vi "Process.vi"(8 "error in":errorcluster, 11 "Qbus in":refnum<class "Qbus.lvclass">) -> (0 "error out":errorcluster)   [LabVIEW 2021, in "AnalogGenerationProcess.lvlib"]
uses:
  AnalogGenerationProcess.lvlib
  <vilib>/addons/Qbus/Qbus.lvclass
  controls/state.ctl
  <vilib>/addons/_NISVFA/_Generation/Signal Generation/SV Signal/SV Signal.lvclass
  controls/generation status.ctl
  <vilib>/addons/_NISVFA/_Generation/Signal Generation/SV Signal/sv_System Timing Model.ctl
  controls/analog generation settings.ctl
  controls/analog output settings.ctl
  controls/terminal configuration.ctl
  controls/signal settings.ctl
  controls/signal type.ctl
  controls/sine wave properties.ctl
  <vilib>/DAQmx/write.llb/DAQmx Write (Analog Wfm 1Chan NSamp).vi
  <vilib>/addons/_NISVFA/_Generation/Signal Generation/SV Sinusoid/SV Sinusoid.lvclass
  C:/Program Files/National Instruments/LabVIEW 2021/vi.lib/addons/_NISVFA/_Generation/Signal Generation/SV Signal/SV Signal.lvclass
  <vilib>/addons/_NISVFA/_Generation/Signal Generation/SV Sinusoid/Configure Sine.vi
  <vilib>/addons/_NISVFA/_Generation/Signal Generation/SV Signal/Write Sample Rate.vi
  <vilib>/addons/_NISVFA/_Generation/Signal Generation/SV Signal/Write System Timing Model.vi
  <vilib>/addons/_NISVFA/_Generation/Signal Generation/SV Signal/Write Ramp Parameters.vi
  <vilib>/DAQmx/miscellaneous.llb/DAQmx Fill In Error Info.vi
  subVIs/utility/AudioGenUtility.lvlib
  shared/logger process/EventLoggerProcess.lvlib
  controls/AudioGenTypeDefs.lvlib
  C:/Program Files/National Instruments/LabVIEW 2021/vi.lib/addons/_NISVFA/_Generation/Signal Generation/SV Function/SV Function.lvclass
  C:/Program Files/National Instruments/LabVIEW 2021/vi.lib/addons/_NISVFA/_Generation/Signal Generation/SV Sinusoid/SV Sinusoid.lvclass
  controls/update signal settings.ctl
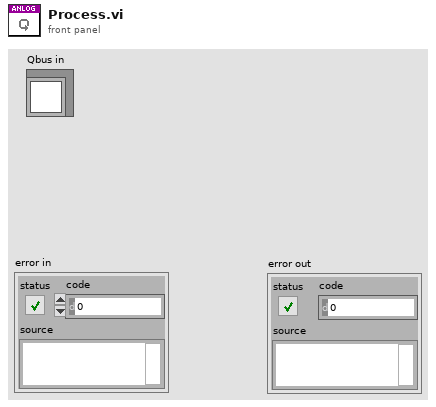
[diagram p1: front panel]
types:
  T1 = typedef "AnalogGenerationProcess.lvlib/state.ctl" = cluster{"DAQmx task":refnum<k21>, "signal configuration":refnum<class "SV Signal.lvclass">, "status":T2}
  T2 = typedef "AudioGenTypeDefs.lvlib/generation status.ctl" = enum16{"Idle", "Committed", "Active"}
  T3 = typedef "AudioGenTypeDefs.lvlib/analog generation settings.ctl" = cluster{"channel list":string, "output settings":T4, "signal settings":T6}
  T4 = typedef "AudioGenTypeDefs.lvlib/analog output settings.ctl" = cluster{"output rate":dbl, "range":dbl, "terminal configuration":T5, "output impedance":dbl, "common mode offset":dbl, "pure tone mode":bool}
  T5 = typedef "AudioGenTypeDefs.lvlib/terminal configuration.ctl" = enum32{"Default", "RSE", "Differential", "Pseudodifferential"}
  T6 = typedef "AudioGenTypeDefs.lvlib/signal settings.ctl" = cluster{"signal type":T7, "properties":string}
  T7 = typedef "AudioGenTypeDefs.lvlib/signal type.ctl" = enum16{"Sine", "Square", "Triangle", "White Noise", "Pink Noise", "Periodic Random Noise"}
  T8 = cluster{"profile":enum16{"Linear", "Half cosine"}, "durations [s]":cluster{"ramp-up":dbl, "transition":dbl, "ramp-down":dbl}}
  T9 = typedef "AudioGenTypeDefs.lvlib/sine wave properties.ctl" = cluster{"frequency":dbl, "amplitude":dbl, "phase":dbl}
  T10 = typedef "AudioGenTypeDefs.lvlib/update signal settings.ctl" = cluster{"frequency":dbl, "gain":dbl}
  T11 = typedef "SV Signal.lvclass/sv_System Timing Model.ctl" = i64
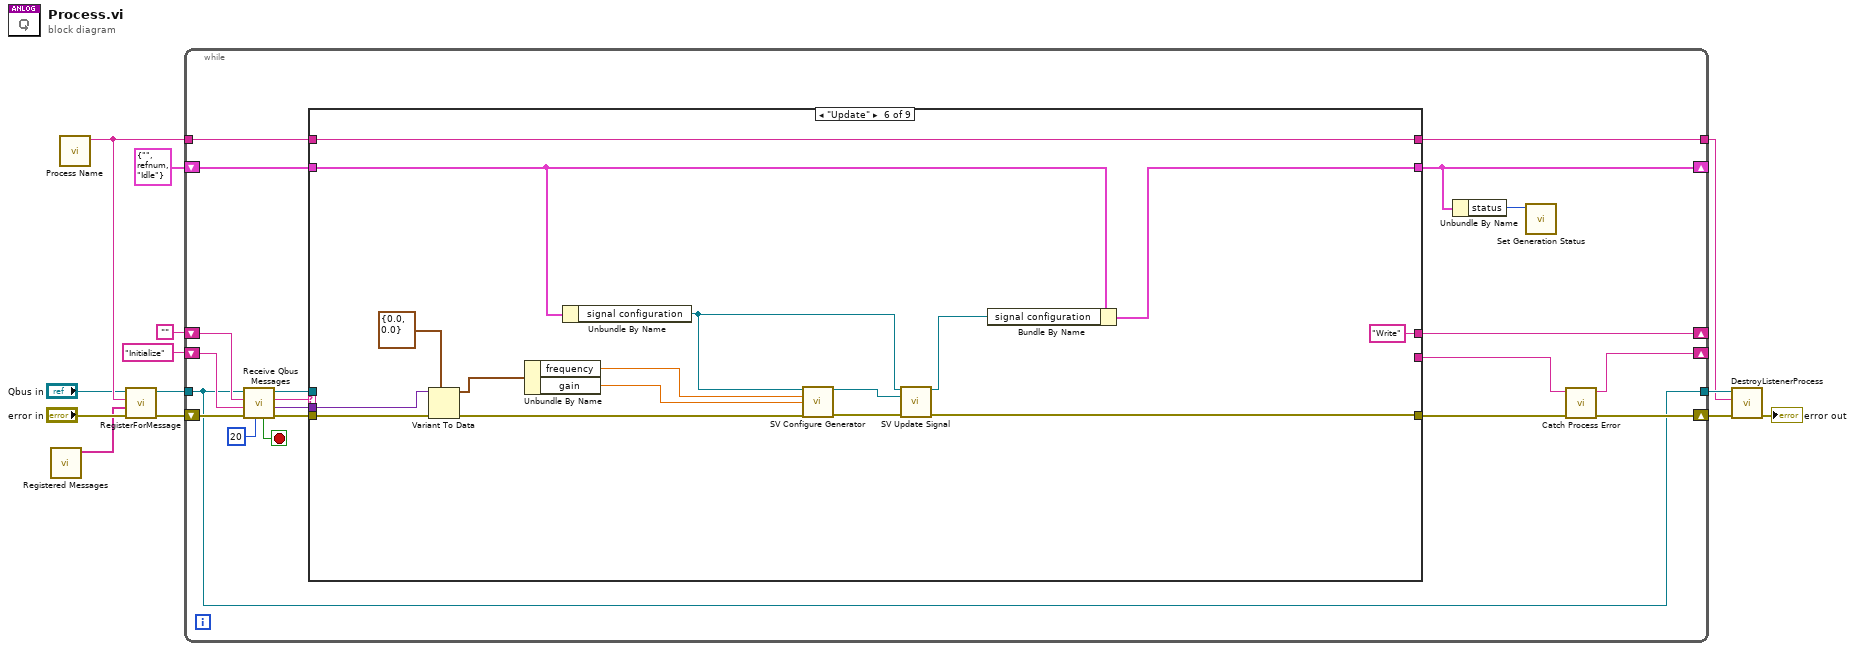
[diagram p0: block diagram]
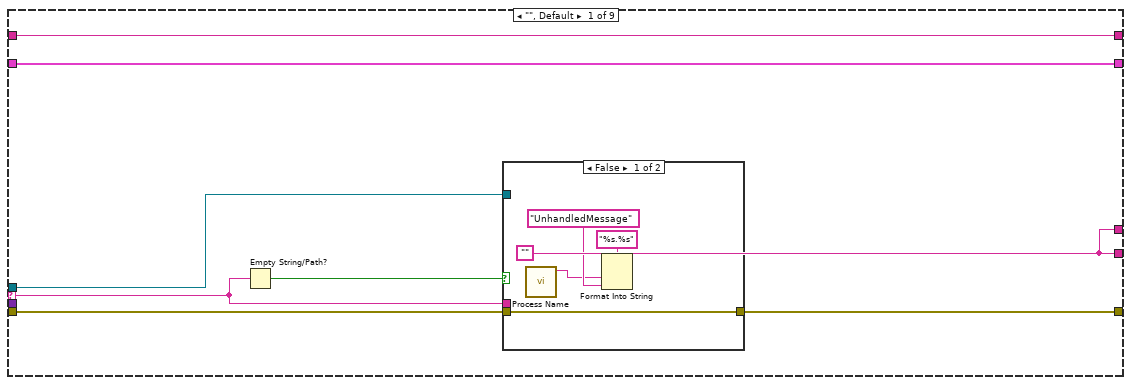
[diagram p2: hidden frame]
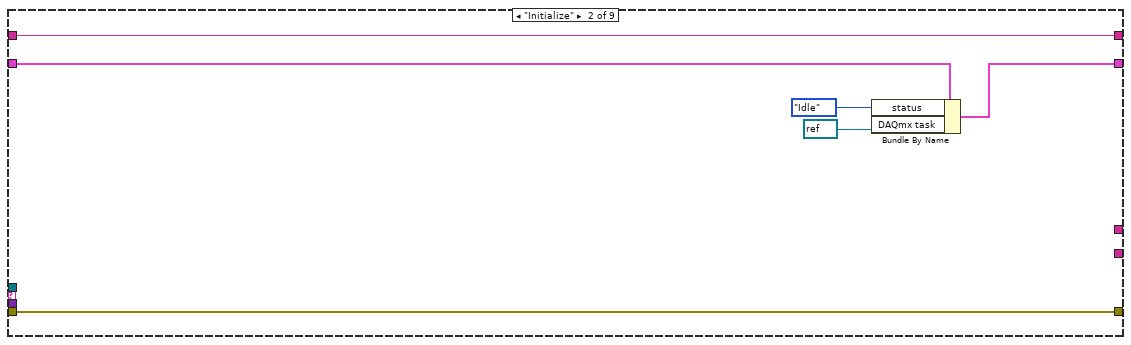
[diagram p4: hidden frame]
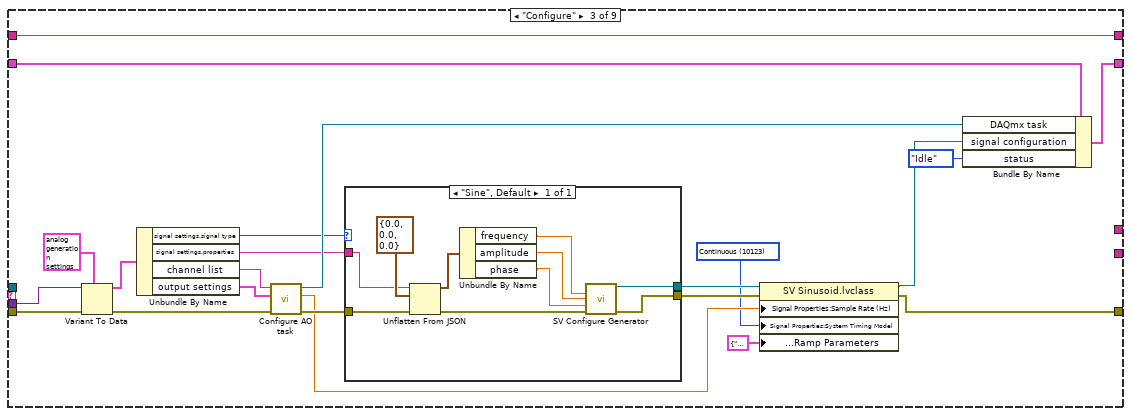
[diagram p5: hidden frame]
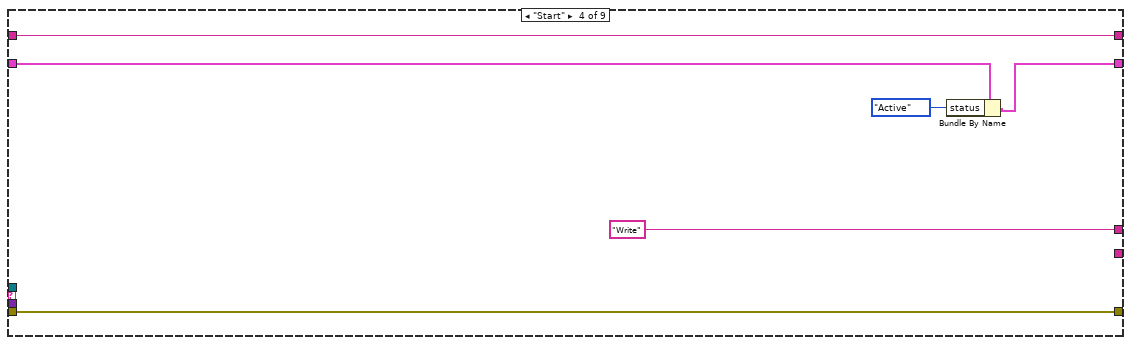
[diagram p6: hidden frame]
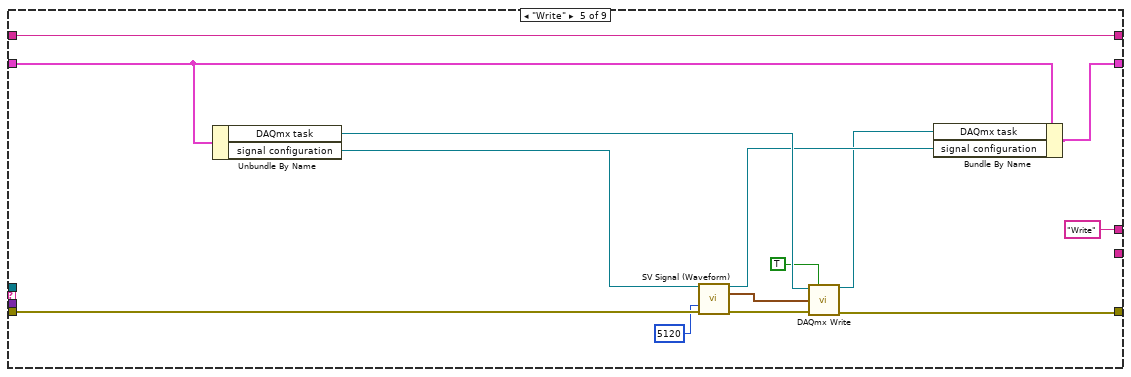
[diagram p7: hidden frame]
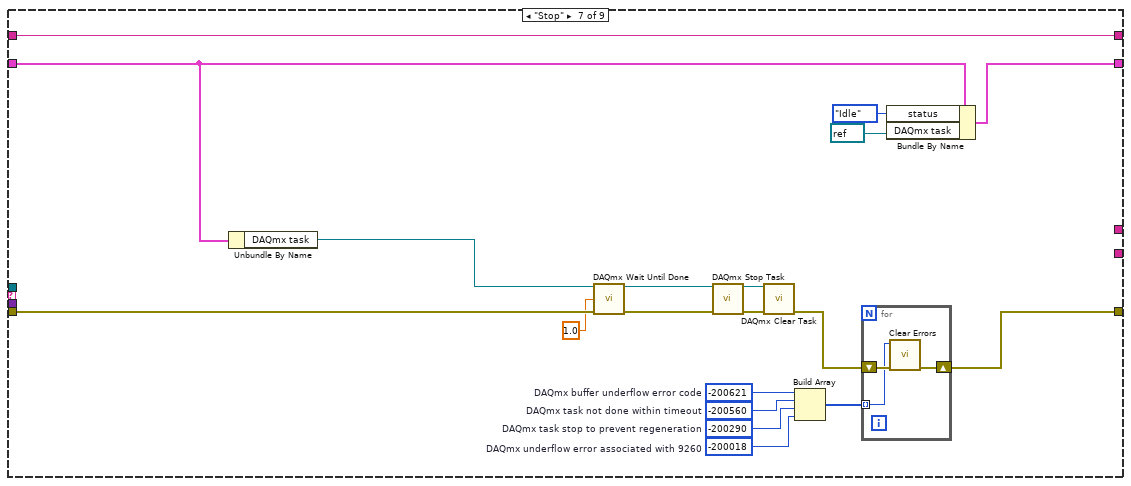
[diagram p8: hidden frame]
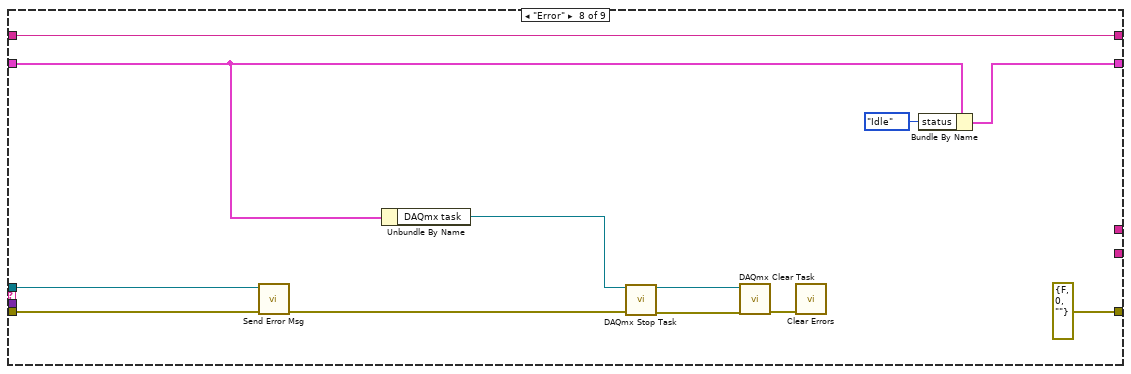
[diagram p9: hidden frame]
diagram:
  n1 = call "Registered Messages.vi"() -> ("registered messages"=w6:string[])  [unwired: 11 in]
  n2 = call "Process Name.vi"() -> ("process name"=w9:string)  [unwired: 11 in]
  n3 = call <vilib>:"RegisterForMessage.vi"("error in (no error)"="error in", "message names"=w6, "process name"=w9, "Qbus in"="Qbus in") -> ("error in (no error)"=w12:errorcluster, "Qbus out"=w13:refnum<class "Qbus.lvclass">)  [unwired: 6 in]
  n4 = while {
    shift-right: [w20] -> _
    shift-left: "" -> [w32]
    tunnel: w13 -> [w16]
    tunnel: w9 -> [w18]
    tunnel: [w16] -> w4
    tunnel: [w22] -> w2
    shift-right: [w26] -> _
    shift-left: "Initialize" -> [w28]
    shift-right: [w27] -> w5
    shift-left: w12 -> [w25]
    shift-right: [w15] -> _
    shift-left: T1 {"DAQmx task"="", "signal configuration"=refnum, "status"=enum."Idle"} ("state") -> [w17]
    stop <- w33 stop-if-true
    n5 = call "Receive Qbus Messages.vi"("timeout(ms)"=20 ("milliseconds to wait"), "error in (no error)"=w25, "priority action"=w28, "default action"=w32, "Qbus in"=w16) -> ("error out"=w31:errorcluster, "message value"=w29:variant, "action"=w24:string, "Qbus out"=w30:refnum<class "Qbus.lvclass">, "exit"=w33:bool)  [unwired: 2 in]
    n6 = case shown="\"Update\"" w24 {
      selector: w24 -> [w38 _ _ _ _ _ _ _ _]
      tunnel: w31 -> [w40 w52 w61 w90 w103 w110 w138 w153 w157]
      tunnel: w30 -> [w36 _ _ _ _ _ _ w152 _]
      tunnel: [w39 w52 w67 w90 w98 w116 w126 errorcluster {"status"=FALSE, "code"=0, "source"=""} ("error out") w157] -> w19
      tunnel: w29 -> [_ _ w62 _ _ w108 _ _ _]
      tunnel: [w41 w51 w74 w89 w104 w120 w139 w154 w156] -> w22
      tunnel: w18 -> [w41 w51 w74 w89 w104 w120 w139 w154 w156]
      tunnel: [w35 _ _ _ _ _ _ _ _] -> w21
      tunnel: [w35 _ _ "Write" "Write" "Write" _ _ _] -> w20
      tunnel: w17 -> [w34 w50 w73 w88 w93 w114 w134 w145 w155]
      tunnel: [w34 w49 w72 w86 w92 w113 w133 w144 w155] -> w15
      frame "", Default {
        w35 = ""
        n7 = Empty String/Path?(string/path=w38) -> (empty?=w37:bool)
        n8 = case shown="False" w37 {
          tunnel: [w42 w46] -> w39
          tunnel: w40 -> [w42 w46]
          tunnel: w38 -> [_ _]
          tunnel: w36 -> [_ _]
          frame False {
            n9 = call "Process Name.vi"() -> ("process name"=w43:string)  [unwired: 11 in]
            n10 = Format Into String(format string="%s.%s", w43, "UnhandledMessage" ("ProcessName")) -> ()  [unwired: 2 in, 2 out]
          }
          frame True {
          }
        }
      }
      frame "Initialize" {
        n11 = Bundle By Name(cluster=w50, "status"=enum16{"Idle", "Committed", "Active"}."Idle", "DAQmx task"=refnum<k21> refnum) -> (w49:T1)
      }
      frame "Configure" {
        w65 = T11 10123 items=["Finite"=10178, "-"=-1, "Continuous"=10123, "-"=-2, "Settled"=110123, "Averaged"=210123, "Discrete Sweep"=310123, "Continuous Sweep"=410123] ("System Timing Model")
        n12 = Variant To Data(error in=w61, type=T3 {"channel list"="", "output settings"={"output rate"=0.0, "range"=0.0, "terminal configuration"=enum."Pseudodifferential", "output impedance"=0.0, "common mode offset"=0.0, "pure tone mode"=FALSE}, "signal settings"={"signal type"=enum."Sine", "properties"=""}} ("analog generation"), Variant=w62) -> (data=w59:T3, error out=w58:errorcluster)
        n13 = Unbundle By Name(w59) -> ("signal settings.signal type"=w57:T7, "signal settings.properties"=w56:string, "channel list"=w55:string, "output settings"=w54:T4)
        n14 = call "Configure AO task.vi"("error in (no error)"=w58, "analog generation"=w54, "physical channels"=w55) -> ("error out"=w71:errorcluster, "actual sample rate"=w66:dbl, "task out"=w63:refnum<k21>)  [unwired: 6 in]
        n15 = case shown="\"Sine\", Default" w57 {
          tunnel: w71 -> [w82]
          tunnel: [w84] -> w70
          tunnel: [w83] -> w69
          tunnel: w56 -> [w79]
          frame "Sine", Default {
            n16 = Unflatten From JSON(JSON string=w79, type and defaults=T9 {"frequency"=0.0, "amplitude"=0.0, "phase"=0.0} ("sine wave properties"), error in (no error)=w82) -> (value=w78:T9, error out=w81:errorcluster)  [unwired: 4 in]
            n17 = Unbundle By Name(w78) -> ("frequency"=w77:dbl, "amplitude"=w76:dbl, "phase"=w75:dbl)
            n18 = call-poly <vilib>:"SV Configure Generator.vi"("frequency (Hz)"=w77, "amplitude"=w76, "phase (deg)"=w75, "error in (no error)"=w81) -> ("signal configuration"=w84:refnum<class "SV Sinusoid.lvclass">, "error out"=w83:errorcluster)  [unwired: 10 in]
          }
        }
        n19 = property class="SV Sinusoid.lvclass"(reference=w70, error in=w69, "Signal Properties:Sample Rate (Hz)"=w66, "Signal Properties:System Timing Model"=w65, "Signal Properties:Ramps:Ramp Parameters"=T8 {"profile"=enum."Half cosine", "durations [s]"={"ramp-up"=0.01, "transition"=0.01, "ramp-down"=0.01}} ("Ramp Parameters:All Elements")) -> (reference out=w68:refnum<class "SV Sinusoid.lvclass">, error out=w67:errorcluster)
        n20 = Bundle By Name(cluster=w73, "DAQmx task"=w63, "signal configuration"=w68, "status"=generation_status."Idle") -> (w72:T1)
      }
      frame "Start" {
        n21 = Bundle By Name(cluster=w88, "status"=enum16{"Idle", "Committed", "Active"}."Active") -> (w86:T1)
      }
      frame "Write" {
        n22 = Unbundle By Name(w93) -> ("DAQmx task"=w100:refnum<k21>, "signal configuration"=w102:refnum<class "SV Signal.lvclass">)
        n23 = call-dynamic "SV Signal (Waveform).vi"("signal configuration"=w102, "samples"=5120, "error in (no error)"=w103) -> ("signal configuration"=w95:refnum<class "SV Signal.lvclass">, "output waveform"=w99:waveform(dbl), "error out"=w101:errorcluster)  [unwired: 7 in, 3 out]
        n24 = call-poly <vilib>:"DAQmx Write.vi"("task/channels in"=w100, "auto start"=TRUE, "data"=w99, "error in"=w101) -> ("task out"=w94:refnum<k21>, "error out"=w98:errorcluster)  [unwired: 9 in, 1 out]
        n25 = Bundle By Name(cluster=w93, "DAQmx task"=w94, "signal configuration"=w95) -> (w92:T1)
      }
      frame "Update" {
        n26 = Variant To Data(error in=w110, type=T10 {"frequency"=0.0, "gain"=0.0} ("signal update setting"), Variant=w108) -> (data=w107:T10, error out=w109:errorcluster)
        n27 = Unbundle By Name(w107) -> ("frequency"=w106:dbl, "gain"=w105:dbl)
        n28 = Unbundle By Name(w114) -> ("signal configuration"=w119:refnum<class "SV Signal.lvclass">)
        n29 = call-poly <vilib>:"SV Configure Generator.vi"("template configuration"=w119, "frequency (Hz)"=w106, "amplitude"=w105, "error in (no error)"=w109) -> ("signal configuration"=w118:refnum<class "SV Sinusoid.lvclass">, "error out"=w117:errorcluster)  [unwired: 10 in]
        n30 = call-dynamic "SV Update Signal.vi"("current configuration"=w119, "new configuration"=w118, "error in"=w117) -> ("updated configuration"=w115:refnum<class "SV Sinusoid.lvclass">, "error out"=w116:errorcluster)  [unwired: 11 in]
        n31 = Bundle By Name(cluster=w114, "signal configuration"=w115) -> (w113:T1)
      }
      frame "Stop" {
        w129 = -200018  # DAQmx underflow error associated with 9260
        w130 = -200290  # DAQmx task stop to prevent regeneration
        w131 = -200560  # DAQmx task not done within timeout
        w132 = -200621  # DAQmx buffer underflow error code
        n32 = Unbundle By Name(w134) -> ("DAQmx task"=w137:refnum<k21>)
        n33 = call <vilib>:"DAQmx Wait Until Done.vi"("task/channels in"=w137, "timeout (sec)"=1.0, "error in"=w138) -> ("task out"=w136:refnum<k21>, "error out"=w127:errorcluster)  [unwired: 11 in]
        n34 = call <vilib>:"DAQmx Stop Task.vi"("task/channels in"=w136, "error in"=w127) -> ("task out"=w124:refnum<k21>, "error out"=w123:errorcluster)  [unwired: 12 in]
        n35 = call <vilib>:"DAQmx Clear Task.vi"("task in"=w124, "error in"=w123) -> ("error out"=w122:errorcluster)  [unwired: 13 in]
        n36 = Build Array(w132, w131, w130, w129) -> (w128:i32[])
        n37 = for {
          shift-right: [w141] -> w126
          shift-left: w122 -> [w142]
          tunnel: w128 -> [w140] mode=indexing
          n38 = call <vilib>:"Clear Errors.vi"("error in (no error)"=w142, "specific error code to clear (0: all)"=w140) -> ("error out"=w141:errorcluster)  [unwired: 4 in, 1 out]
        }
        n39 = Bundle By Name(cluster=w134, "status"=generation_status."Idle", "DAQmx task"=refnum<k21> refnum) -> (w133:T1)
      }
      frame "Error" {
        n40 = call "Send Error Msg.vi"("error in"=w153, "Qbus in"=w152) -> ("error out"=w150:errorcluster)  [unwired: 8 in, 1 out]
        n41 = Unbundle By Name(w145) -> ("DAQmx task"=w149:refnum<k21>)
        n42 = call <vilib>:"DAQmx Stop Task.vi"("task/channels in"=w149, "error in"=w150) -> ("task out"=w148:refnum<k21>, "error out"=w147:errorcluster)  [unwired: 12 in]
        n43 = call <vilib>:"DAQmx Clear Task.vi"("task in"=w148, "error in"=w147) -> ("error out"=w146:errorcluster)  [unwired: 13 in]
        n44 = call <vilib>:"Clear Errors.vi"("error in (no error)"=w146) -> ()  [unwired: 5 in, 2 out]
        n45 = Bundle By Name(cluster=w145, "status"=generation_status."Idle") -> (w144:T1)
      }
      frame "Exit" {
      }
    }
    n46 = Unbundle By Name(w15) -> ("status"=w14:T2)
    n47 = call "Set Generation Status.vi"("status"=w14) -> ()  [unwired: 10 in, 1 out]
    n48 = call "Catch Process Error.vi"("error in (no error)"=w19, "priority action"=w21) -> ("error out"=w27:errorcluster, "priority action"=w26:string)  [unwired: 8 in]
  }
  n49 = call <vilib>:"DestroyListenerProcess.vi"("error in (no error)"=w5, "process name"=w2, "Qbus in"=w4) -> ("error in (no error)"=→"error out":errorcluster)  [unwired: 7 in, 1 out]
